vi "hMediBtnController.vi"(7 "state":enum16{"Init", "enable"}(ring), 8 "error in (no error)":errorcluster caption="에러 입력(에러 없음)", 10 "2dArray":string[][](table), 11 "btnGroup":refnum<vi>) -> (0 "error out":errorcluster caption="에러 출력")   [LabVIEW 2019]
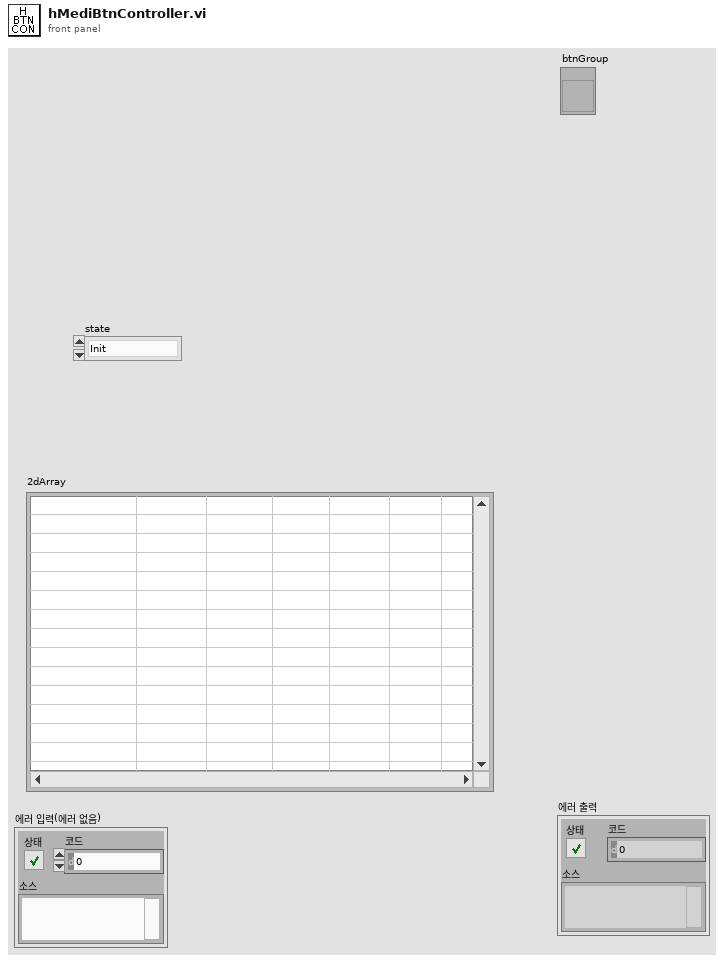
[diagram p1: front panel]
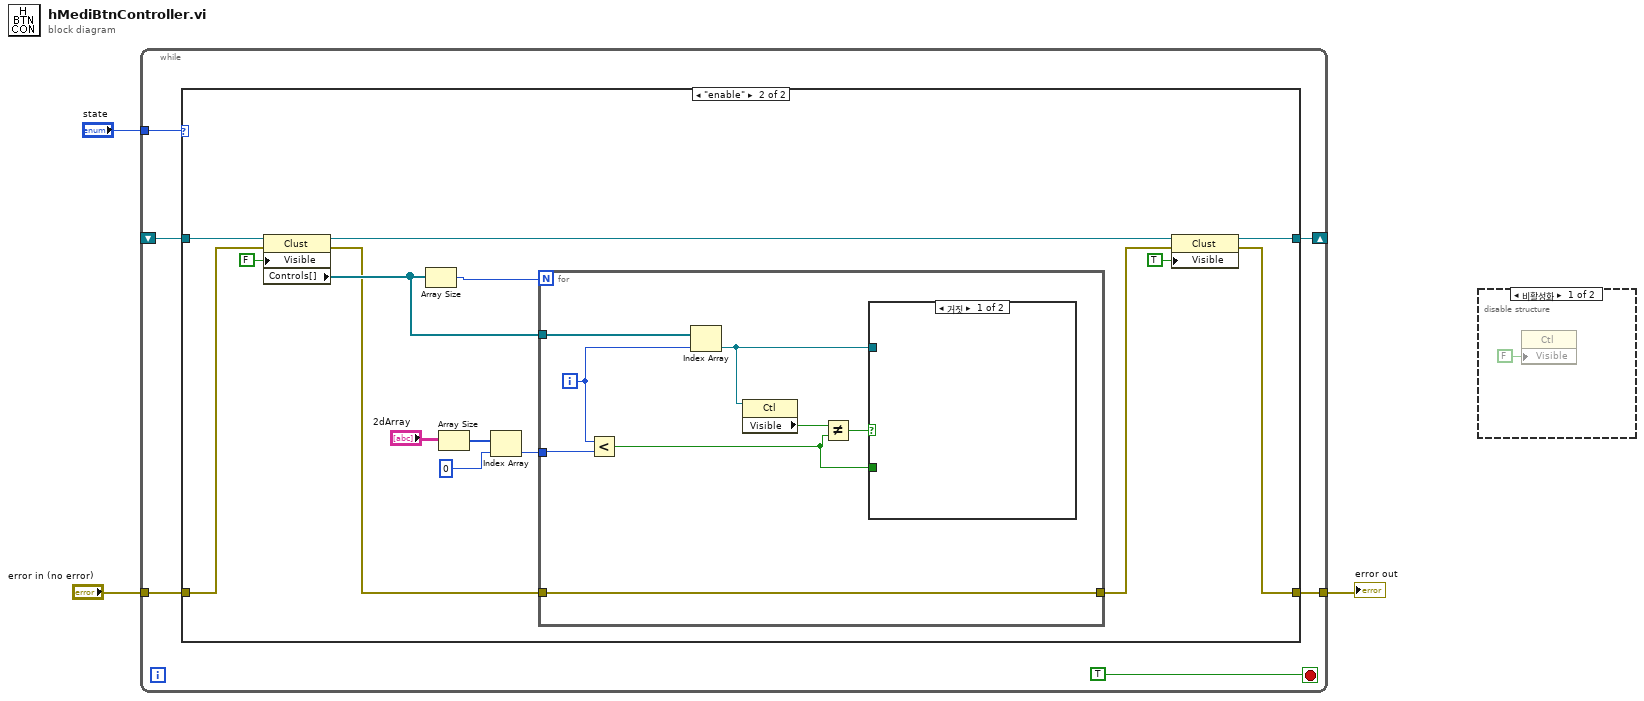
[diagram p0: block diagram]
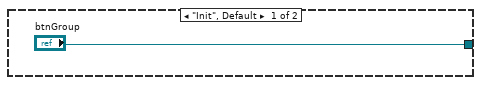
[diagram p3: hidden frame]
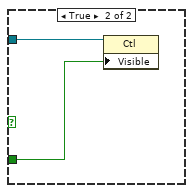
[diagram p4: hidden frame]
diagram:
  n1 = while {
    tunnel: "state" -> [w9]
    shift-right: [w8] -> _
    shift-left: _ -> [w7]
    tunnel: "error in (no error)" -> [w5]
    tunnel: [w4] -> w1
    stop <- TRUE stop-if-true
    n2 = case shown="\"enable\"" w9 {
      tunnel: ["btnGroup" w15] -> w8
      tunnel: w7 -> [_ w16]
      tunnel: w5 -> [_ w17]
      tunnel: [_ w13] -> w4
      frame "Init", Default {
      }
      frame "enable" {
        n3 = property class="Clust"(reference=w16, error in=w17, "Visible"=FALSE ("보이기")) -> (error out=w18:errorcluster, "Controls[]"=w20:refnum<vi>[])  [unwired: 1 out]
        n4 = Array Size(array=w20) -> (size(s)=w11:i32)
        n5 = Array Size(array="2dArray") -> (size(s)=w23:i32[])
        n6 = Index Array(array=w23, index=0 ("인덱스")) -> (element=w21:i32)
        n7 = for {
          N: w11 -> [_]
          tunnel: w21 -> [w32]
          tunnel: w20 -> [w27]
          tunnel: w18 -> [w26]
          tunnel: [w26] -> w14
          i -> [w25]
          n8 = Less?(x=w25, y=w32) -> (x < y?=w28:bool)
          n9 = Index Array(array=w27, index=w25) -> (element=w31:refnum<vi>)
          n10 = property class="Ctl"(reference=w31) -> ("Visible"=w30:bool)  [unwired: 1 in, 2 out]
          n11 = Not Equal?(x=w30, y=w28) -> (x != y?=w29:bool)
          n12 = case shown="거짓" w29 {
            tunnel: w31 -> [_ w34]
            tunnel: w28 -> [_ w33]
            frame False {
            }
            frame True {
              n13 = property class="Ctl"(reference=w34, "Visible"=w33) -> ()  [unwired: 1 in, 2 out]
            }
          }
        }
        n14 = property class="Clust"(reference=w16, error in=w14, "Visible"=TRUE ("보이기")) -> (reference out=w15:refnum<vi>, error out=w13:errorcluster)
      }
    }
  }
  "error out" <- w1
  n15 = disable-structure shown="비활성화" {
    frame Disabled {
      n16 = property class="Ctl"("Visible"=FALSE ("보이기")) -> ()  [unwired: 2 in, 2 out]
    }
    frame Enabled {
    }
  }
